vi "HelloWorld.vi"(8 "error in (no error)":errorcluster, 11 "Actor 1 - State machine in":refnum<class "Actor 1 - State machine.lvclass">) -> (0 "error out":errorcluster, 3 "Actor 1 - State machine out":refnum<class "Actor 1 - State machine.lvclass">)   [LabVIEW 2020, in "Actor 1 - State machine.lvlib" / "Actor 1 - State machine.lvclass"]
uses:
  Actor 1 - State machine.lvclass
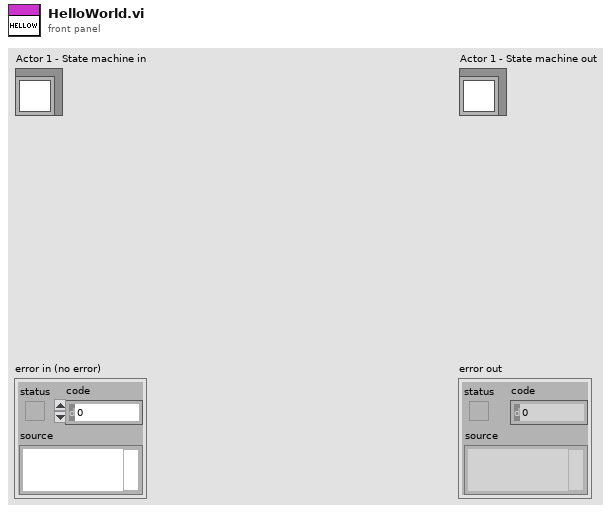
[diagram p1: front panel]
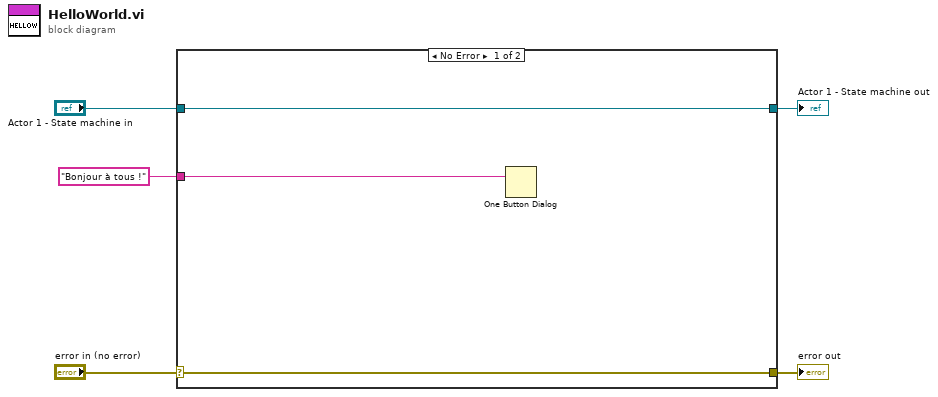
[diagram p0: block diagram]
diagram:
  n1 = case shown="No Error" "error in (no error)" {
    selector: "error in (no error)" -> [w7 w10]
    tunnel: [w7 w10] -> w4
    tunnel: [w8 w9] -> w2
    tunnel: "Actor 1 - State machine in" -> [w8 w9]
    tunnel: "Bonjour à tous !" ("message") -> [w6 _]
    frame No Error {
      n2 = One Button Dialog(message=w6) -> ()  [unwired: 1 in, 1 out]
    }
    frame Error {
    }
  }
  "error out" <- w4
  "Actor 1 - State machine out" <- w2
